vi "Create Tree Tag.vi"(10 "WID":string, 11 "DC_UID":T1) -> (3 "Tree Tag":string)   [LabVIEW 2017, in "Application Manager.lvclass"]
doc: "Create unique tag for item in tree"
uses:
  Application Manager.lvclass
  Common VIs/DC_UID.ctl
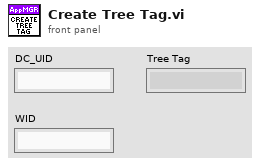
[diagram p1: front panel]
types:
  T1 = typedef "DC_UID.ctl" = string
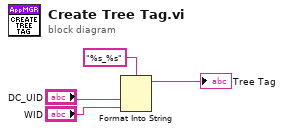
[diagram p0: block diagram]
diagram:
  n1 = Format Into String(format string="%s_%s", "DC_UID", "WID") -> (resulting string=→"Tree Tag":string)  [unwired: 2 in, 1 out]
